vi "Initialize.vi"(8 "error in":errorcluster, 10 "parameters":variant, 11 "Digitizer Channel in":refnum<class "Digitizer Channel.lvclass">) -> (0 "error out":errorcluster, 2 "summary":T2[](array[typedef]), 3 "data value reference":T1)   [LabVIEW 2025, in "Digitizer.lvlib" / "Digitizer Channel.lvclass"]
doc: "This Vi initializes the data of a node its default state.\nThe object is not created inside of this ViI, beacuase it is created from a File depending on user selection.Copyright 2017 National Instruments Corporation\n\nLicensed under the Apache License, Version 2.0 (the \"License\"); you may not use this file except in compliance with the License. You may obtain a copy of the License at http://www.apache.org/licenses/LICENSE-2.0\nUnless required by applicable law or agreed to in writing, software distributed under the License is distributed on an \"AS IS\" BASIS, WITHOUT WARRANTIES OR CONDITIONS OF ANY KIND, either express or implied. See the License for the specific language governing permissions and limitations under the License."
uses:
  Digitizer Channel.lvclass
  C:/Users/Public/Documents/Sandia National Labs/TSS Plugin/CEF.lvlibp/Node/CEF_Node.lvclass
  Users/Public/Documents/Sandia National Labs/TSS Plugin/CEF.lvlibp/Node/Summary.ctl
  Users/Public/Documents/Sandia National Labs/TSS Plugin/CEF.lvlibp/Node/NodeRef.ctl
  Users/Public/Documents/Sandia National Labs/TSS Plugin/CEF.lvlibp/Node/CEF_Node.lvclass
  Digitizer Instrument/Digitizer Instrument.lvclass
  Digitizer Channel.lvclass/Digitizer Channel.ctl
  Digitizer configuration/Digitizer configuration.lvclass
  C:/Users/Public/Documents/Sandia National Labs/TSS Plugin/Abstract Engine.lvlibp/Instrument configuration/Instrument configuration.lvclass
  Digitizer Channel configuration/Digitizer Channel configuration.lvclass
  C:/Users/Public/Documents/Sandia National Labs/TSS Plugin/Abstract Engine.lvlibp/Channel configuration/Channel configuration.lvclass
  Users/Public/Documents/Sandia National Labs/TSS Plugin/CEF.lvlibp/Node/ReadParent.vi
  Users/Public/Documents/Sandia National Labs/TSS Plugin/CEF.lvlibp/Node/ReadChildren.vi
  Users/Public/Documents/Sandia National Labs/TSS Plugin/Abstract Engine.lvlibp/Instrument configuration/Read Instrument Setting.vi
  Users/Public/Documents/Sandia National Labs/TSS Plugin/Abstract Engine.lvlibp/Channel configuration/Read Channel Setting.vi
  Users/Public/Documents/Sandia National Labs/TSS Plugin/Abstract Engine.lvlibp/Channel configuration/Write Channel Setting.vi
  Users/Public/Documents/Sandia National Labs/TSS Plugin/CEF.lvlibp/serializable configuration/CEF_serializable configuration.lvclass
  Users/Public/Documents/Sandia National Labs/TSS Plugin/Abstract Engine.lvlibp/Abstract Channel/Abstract Channel.lvclass
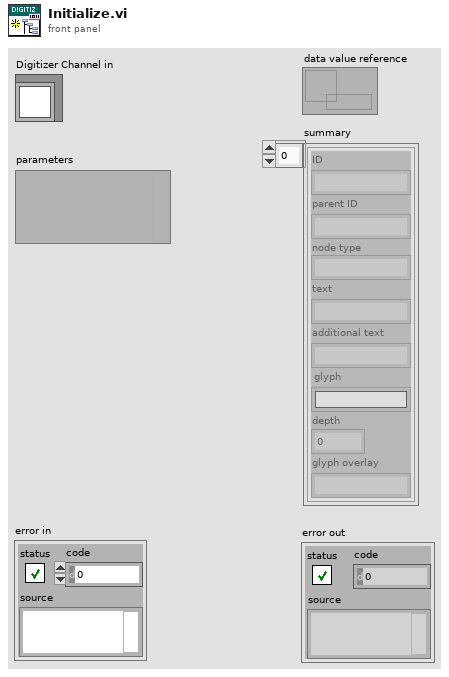
[diagram p1: front panel]
types:
  T1 = typedef "CEF.lvlibp/CEF_Node.lvclass/NodeRef.ctl" = refnum<data-value>
  T2 = typedef "CEF.lvlibp/CEF_Node.lvclass/Summary.ctl" = cluster{"ID":string, "parent ID":string, "node type":string, "text":string, "additional text":string, "glyph":string, "depth":i32, "glyph overlay":string}
  T3 = typedef "Abstract Engine.lvlibp/Instrument configuration.lvclass/Default Instrument.ctl" = cluster{"Type":string, "Address":string, "SW Alias":string, "Description":string, "Enabled":bool}
  T4 = typedef "Abstract Engine.lvlibp/Channel configuration.lvclass/Default Channel.ctl" = cluster{"Address":string, "SW Alias":string, "Enabled":bool, "Type":string, "Description":string}
  T5 = cluster{"ID":string, "parent ID":string, "node type":string, "text":string, "additional text":string, "glyph":string, "depth":i32, "glyph overlay":string}[]
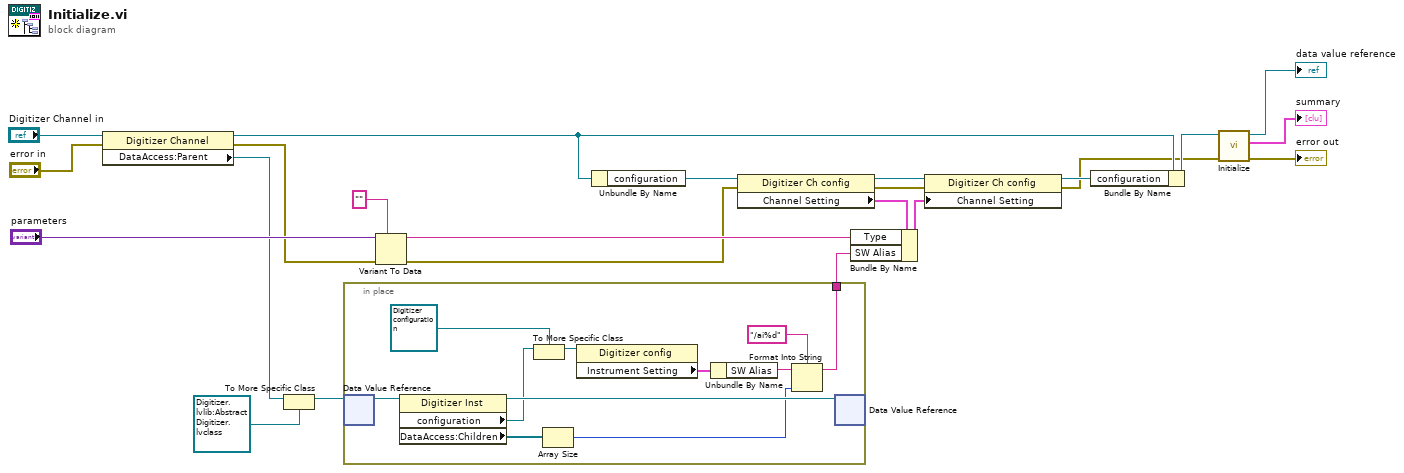
[diagram p0: block diagram]
diagram:
  n1 = property class="Digitizer Channel"(reference="Digitizer Channel in", error in="error in") -> (reference out=w15:refnum<class "Digitizer Channel.lvclass">, error out=w10:errorcluster, "DataAccess:Parent"=w17:refnum<data-value>)
  n2 = To More Specific Class(target class=refnum<data-value> refnum ("data value reference"), reference=w17) -> (specific class reference=w18:refnum<data-value>)  [unwired: 1 in, 1 out]
  n3 = in-place {
    in-place-border: [w32] -> w11
    n4 = in-place-dvr #1(w18) -> (w31:refnum<class "Digitizer Instrument.lvclass">)  [unwired: 1 out]
    n5 = property class="Digitizer Inst"(reference=w31) -> (reference out=w30:refnum<class "Digitizer Instrument.lvclass">, "configuration"=w29:refnum<class "CEF_serializable configuration.lvclass">, "DataAccess:Children"=w28:refnum<data-value>[])  [unwired: 1 in, 1 out]
    n6 = To More Specific Class(target class=refnum<class "Digitizer configuration.lvclass"> refnum ("Digitizer.lvlib:Digitizer configuration.lvclass"), reference=w29) -> (specific class reference=w34:refnum<class "Digitizer configuration.lvclass">)  [unwired: 1 in, 1 out]
    n7 = Array Size(array=w28) -> (size(s)=w26:i32)
    n8 = property class="Digitizer config"(reference=w34) -> ("Instrument Setting"=w25:T3)  [unwired: 1 in, 2 out]
    n9 = Unbundle By Name(w25) -> ("SW Alias"=w33:string)
    n10 = Format Into String(format string="/ai%d", initial string=w33, w26) -> (resulting string=w32:string)  [unwired: 1 in, 1 out]
    n11 = in-place-dvr #1(w30) -> ()  [unwired: 2 out]
  }
  n12 = Variant To Data(error in=w10, type="", Variant="parameters") -> (data=w7:string, error out=w5:errorcluster)
  n13 = Unbundle By Name(w15) -> ("configuration"=w16:refnum<class "Digitizer Channel configuration.lvclass">)
  n14 = property class="Digitizer Ch config"(reference=w16, error in=w5) -> (reference out=w6:refnum<class "Digitizer Channel configuration.lvclass">, error out=w2:errorcluster, "Channel Setting"=w4:T4)
  n15 = Bundle By Name(cluster=w4, "Type"=w7, "SW Alias"=w11) -> (w3:T4)
  n16 = property class="Digitizer Ch config"(reference=w6, error in=w2, "Channel Setting"=w3) -> (reference out=w13:refnum<class "Digitizer Channel configuration.lvclass">, error out=w9:errorcluster)
  n17 = Bundle By Name(cluster=w15, "configuration"=w13) -> (w14:refnum<class "Digitizer Channel.lvclass">)
  n18 = call-parent "Initialize.vi"("error in"=w9, "CEF_Serialize node in"=w14) -> ("error out"=→"error out":errorcluster, "summary"=→"summary":T5, "data value reference"=→"data value reference":refnum<data-value>)  [unwired: 7 in]
